vi "Post.vi"(7 "Datum":refnum<class "Datum.lvclass">, 8 "Error In":errorcluster, 10 "Output In":string, 11 "Mock In":refnum<class "Mock Compile Hook.lvclass">) -> (0 "Error Out":errorcluster, 2 "Output Out":string, 3 "Mock Out":refnum<class "Mock Compile Hook.lvclass">)   [LabVIEW 2018, in "Tests.lvlib" / "Compile.lvlib" / "Mock Compile Hook.lvclass"]
uses:
  Mock Compile Hook.lvclass
  src/Toolkit/Data/Datum/Datum.lvclass
  Mock Compile Hook.lvclass/Mock Compile Hook.ctl
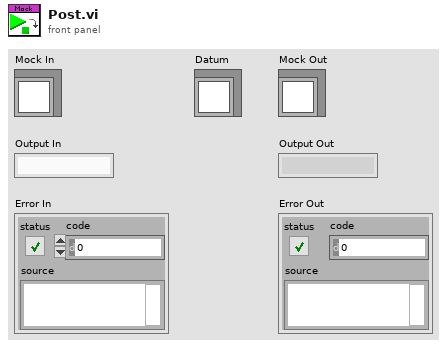
[diagram p1: front panel]
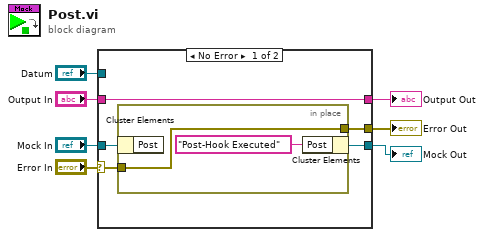
[diagram p0: block diagram]
diagram:
  n1 = case shown="No Error" "Error In" {
    selector: "Error In" -> [w9 w16]
    tunnel: [w8 w16] -> w5
    tunnel: "Output In" -> [w12 _]
    tunnel: [w12 _] -> w6
    tunnel: "Mock In" -> [w11 w15]
    tunnel: [w10 w15] -> w4
    tunnel: "Datum" -> [_ _]
    frame No Error {
      n2 = in-place {
        in-place-border: w9 -> [w13]
        in-place-border: [w13] -> w8
        n3 = in-place-cluster #1(w11) -> ()  [unwired: 1 out]
        n4 = in-place-cluster #1("Post"="Post-Hook Executed" ("Pre")) -> (w10:refnum<class "Mock Compile Hook.lvclass">)
      }
    }
    frame Error {
    }
  }
  "Mock Out" <- w4
  "Error Out" <- w5
  "Output Out" <- w6
